vi "niRFUtil MASMT 1D Cross Correlation (DBL, CDB).vi"(6 "normalization":i32(ring) items=["None", "Unbiased", "Biased"], 8 "error in (no error)":errorcluster, 9 "algorithm":i32(ring)=1 items=["Direct", "Frequency Domain"], 10 "Y":cdb[](array[numeric]), 11 "X":dbl[](array[numeric])) -> (0 "error out":errorcluster, 3 "Rxy":cdb[](array[numeric]))   [LabVIEW 2015, in "niRFUtil.lvlib"]
doc: "Computes the cross correlation of the input sequences <B>X</B> and <B>Y</B>."
uses:
  niRFUtil.lvlib
  Utilities/niRFMASMT_FFT.dll
panel:
  out "FreqWorkH":cdb[](array[numeric])
  out "WorkH":dbl[](array[numeric])
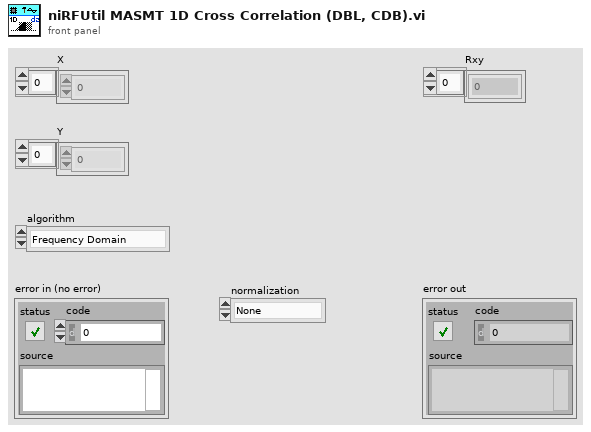
[diagram p1: front panel]
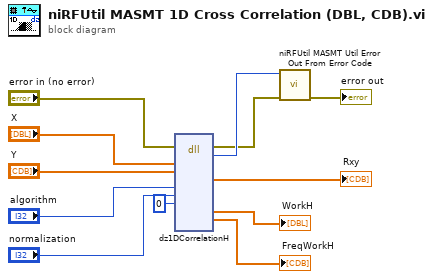
[diagram p0: block diagram]
diagram:
  n1 = dll-call lib="C:/Perforce/semoore-sales/Customers/NATI-3813/Noise Floor/LV Filters/ParallelComplexFilterRFUtil/niRFUtil/MASMT/Utilities/niRFMASMT_FFT.*" fn="dz1DCorrelationH"(error in="error in (no error)", "X"="X", "Y"="Y", "domain"="algorithm", "norm"="normalization", "step"=0) -> (error out=w5:errorcluster, "error"=w7:i32, "Rxy"=→"Rxy":cdb[], "txWorkH"=→"WorkH":dbl[], "FreqWorkH"=→"FreqWorkH":cdb[])  [unwired: 12 in, 1 out]
  n2 = call "niRFUtil MASMT Util Error Out From Error Code.vi"("error in (no error)"=w5, "error code"=w7) -> ("error out"=→"error out":errorcluster)  [unwired: 9 in]
